vi "Update Task Point Data.vi"(7 "Task Ident":string, 8 "error in":errorcluster, 9 "Data":variant, 10 "Point Ident":string, 11 "Series Actor in":refnum<class "Series Actor.lvclass">) -> (0 "error out":errorcluster, 3 "Series Actor out":refnum<class "Series Actor.lvclass">)   [LabVIEW 2023, in "HAL GOOP4.lvlib" / "Series Actor.lvlib" / "Series Actor.lvclass"]
uses:
  Series Actor.lvclass
  Series Actor.lvclass/Series Actor.ctl
  <vilib>/ErrorRing/Error Ring.xnode
  <vilib>/Utility/error.llb/Error Cluster From Error Code.vi
  Task/ITask Actor/ITask Actor Messages/Position Data Updated Msg/Position Data Updated Msg.lvclass
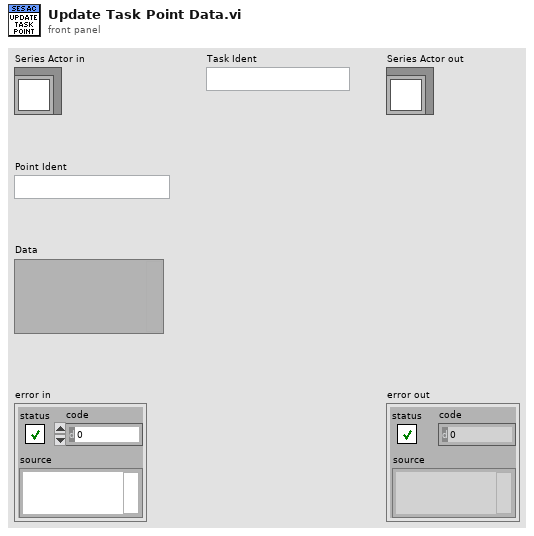
[diagram p1: front panel]
types:
  T1 = map{string, refnum<class "Message Enqueuer.lvclass">}
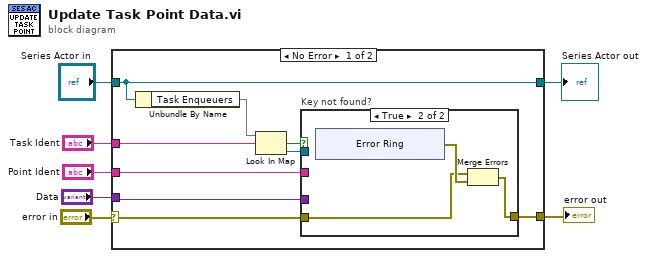
[diagram p0: block diagram]
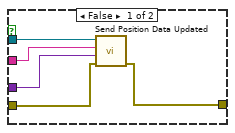
[diagram p2: hidden frame]
diagram:
  n1 = case shown="No Error" "error in" {
    selector: "error in" -> [w11 w30]
    tunnel: [w16 w31] -> w5
    tunnel: "Series Actor in" -> [w16 w31]
    tunnel: "Task Ident" -> [w14 _]
    tunnel: "Point Ident" -> [w10 _]
    tunnel: "Data" -> [w9 _]
    tunnel: [w8 w30] -> w1
    frame No Error {
      n2 = Unbundle By Name(w16) -> ("Task Enqueuers"=w15:T1)
      n3 = Look In Map(map=w15, key=w14) -> (key not found?=w13:bool, value=w12:refnum<class "Message Enqueuer.lvclass">)  [unwired: 1 in]
      n4 = case "Key not found?" shown="True" w13 {
        tunnel: w12 -> [w21 _]
        tunnel: w11 -> [w18 w23]
        tunnel: w10 -> [w20 _]
        tunnel: w9 -> [w19 _]
        tunnel: [w17 w22] -> w8
        frame False {
          n5 = call "Send Position Data Updated.vi"("error in (no error)"=w18, "Data"=w19, "Point Ident"=w20, "Message Enqueuer"=w21) -> ("error out"=w17:errorcluster)  [unwired: 6 in, 1 out]
        }
        frame True {
          n6 = xnode "Error Ring"() -> ("error out"=w24:errorcluster)
          n7 = Merge Errors(w23, w24) -> (w22:errorcluster)
        }
      }
    }
    frame Error {
    }
  }
  "error out" <- w1
  "Series Actor out" <- w5
